vi "UNITTESTS.vi"   [LabVIEW 2019]
uses:
  <vilib>/addons/_JKI Toolkits/Caraya/classes/Test/Test.lvclass
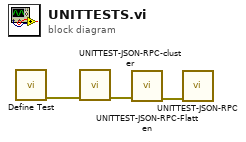
[diagram p0: block diagram]
diagram:
  n1 = call <vilib>:"Define Test.vi"() -> ("error out"=w2:errorcluster)  [unwired: 10 in, 1 out]
  n2 = call "UNITTEST-JSON-RPC-cluster.vi"("error in (no error)"=w2) -> ("error out"=w3:errorcluster)  [unwired: 10 in]
  n3 = call "UNITTEST-JSON-RPC-Flatten.vi"("error in (no error)"=w3) -> ("error out"=w1:errorcluster)  [unwired: 10 in]
  n4 = call "UNITTEST-JSON-RPC.vi"("error in (no error)"=w1) -> ()  [unwired: 10 in, 1 out]
